vi "R(T) T(t) SETP(t) with ramp332 DC ramp current(File overwrite Fixed)_1.vi"(0 "I":dbl=1e-06 min=1e-09 max=1.0 step=1e-06 format="%.4e", 1 "Ti":dbl min=0.0 max=400.0 format="%.3f", 2 "Tf":dbl=4.0 min=0.0 max=400.0 format="%.3f", 3 "Ramp":ext format="%.3f", 4 "Range":dbl=3.0 format="%.2f", 7 "Measurement":bool=TRUE, 8 "Auto\nTemp?":bool=TRUE) -> ()   [LabVIEW 2012]
panel:
  out "?":cluster{dbl, dbl}[](graph)
  out "?":cluster{"X":dbl, "Y":dbl}[](graph)
  in  "x data precision":i16
  in  "y data precision":i16
  in  "Path":path
  in  "File name":string
  in  "Autorange":bool=TRUE
  in  "Volt Delay":u32=50
  in  "Voltmeter PLC":dbl=1.0 min=0.01 max=60.0 step=0.01 format="%.2f"
  in  "Voltage Compliance":dbl=12.0 min=0.1 max=105.0 step=0.1 format="%.2f"
  in  "minutes to wait before start":u32=5
  out "R/Ohm":dbl=1e-09 min=-1.0 step=1e-09 format="%.3e"
  out "T/K":dbl min=0.0 step=0.01 format="%.3f"
  in  "Delay time":sgl min=0 step=1 format="%.2f"
  # "ON"
  # "OFF"
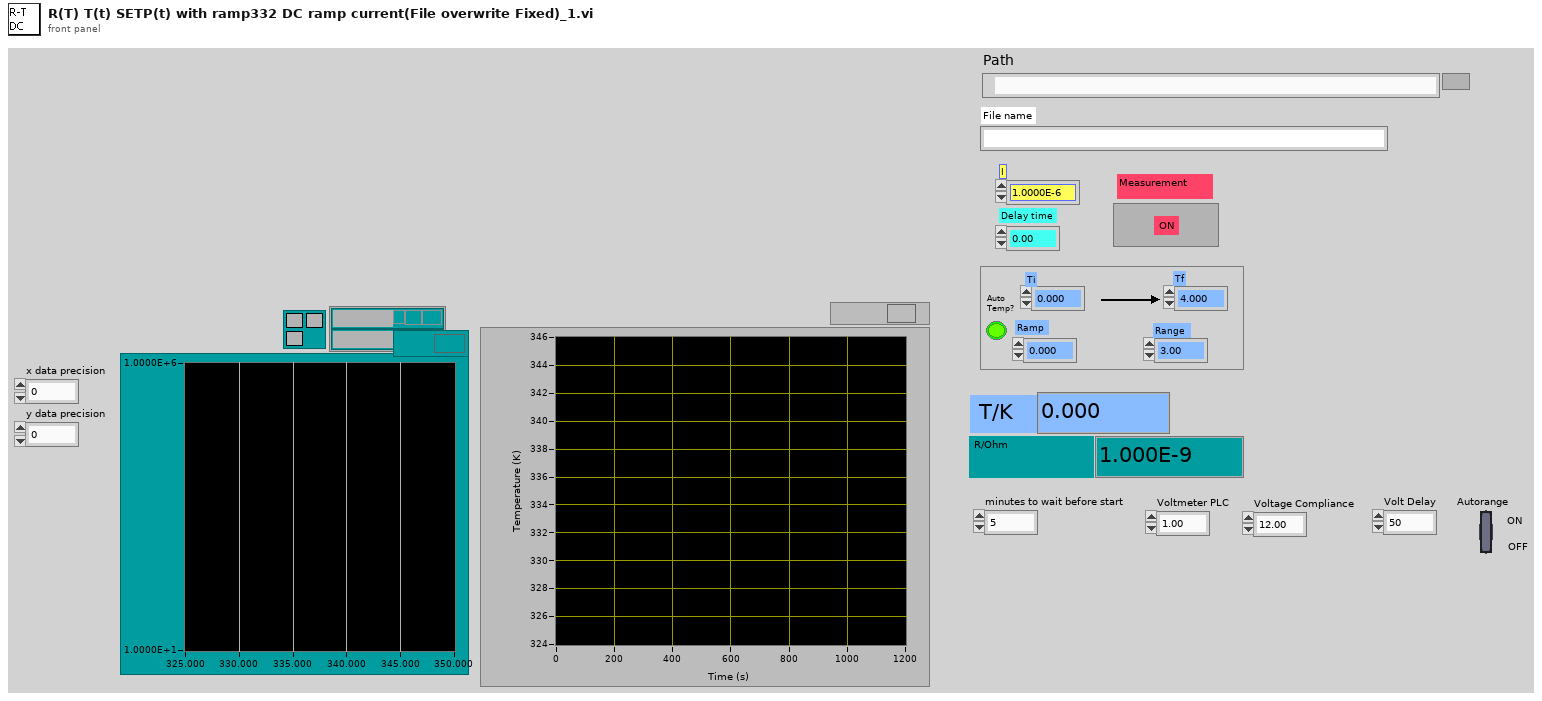
[diagram p1: front panel]
types:
  T1 = enum16{"open", "replace", "create", "open or create", "replace or create", "replace or create with confirmation"}
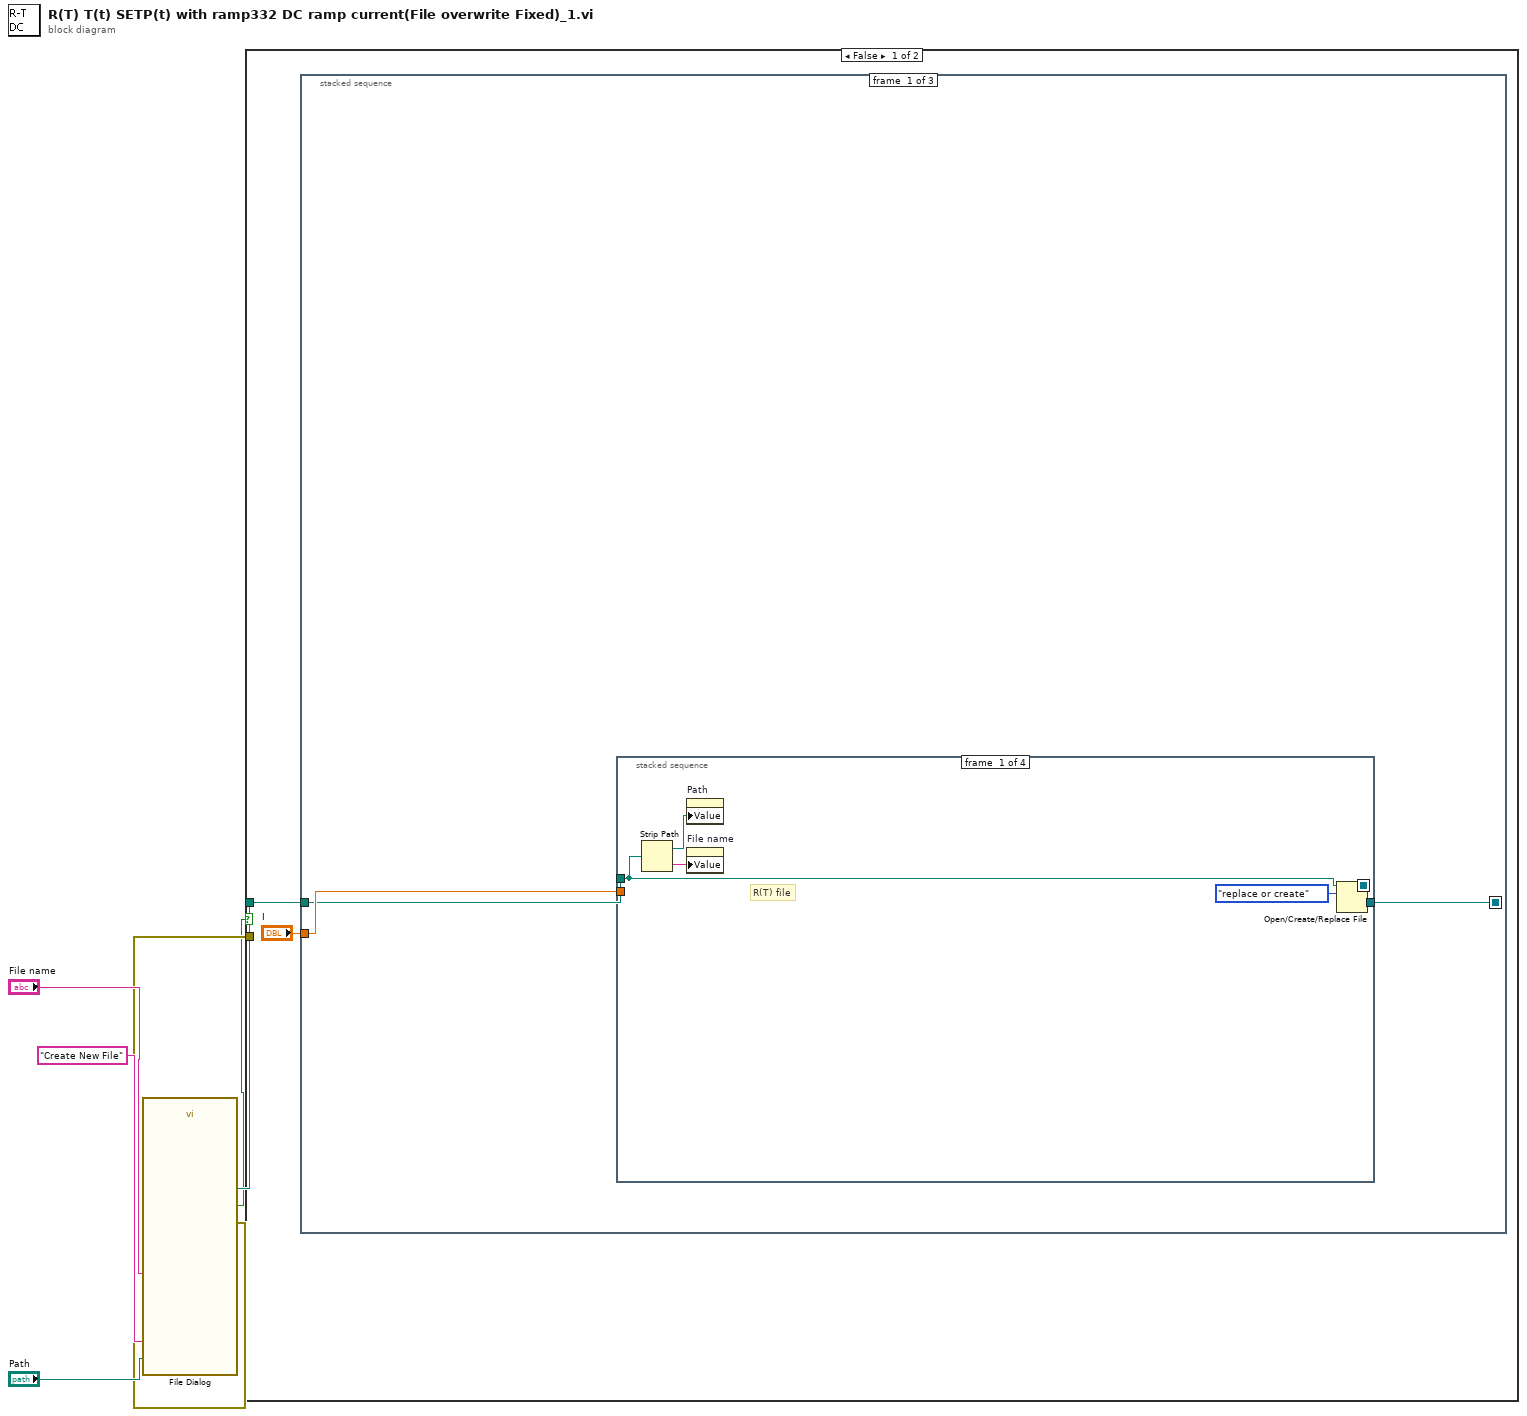
[diagram p0: block diagram]
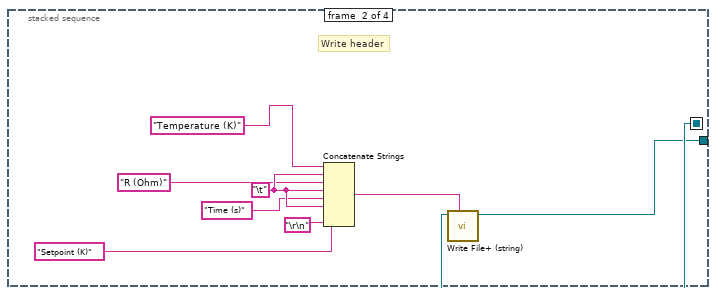
[diagram p2: hidden frame]
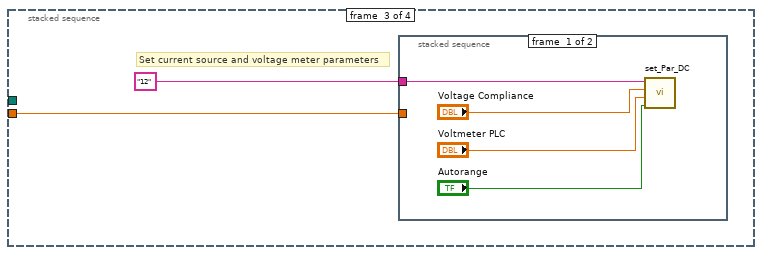
[diagram p3: hidden frame]
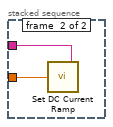
[diagram p4: hidden frame]
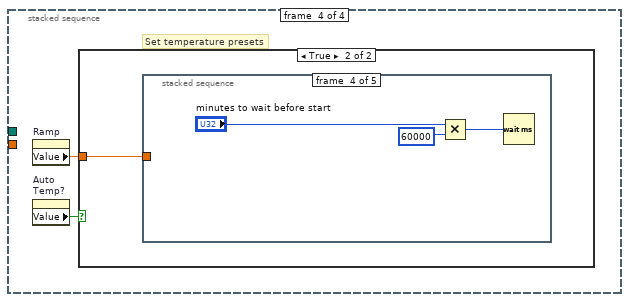
[diagram p5: hidden frame]
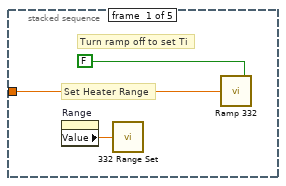
[diagram p7: hidden frame]
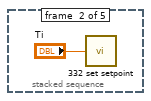
[diagram p8: hidden frame]
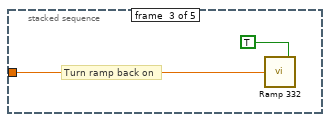
[diagram p9: hidden frame]
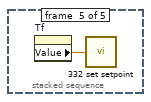
[diagram p10: hidden frame]
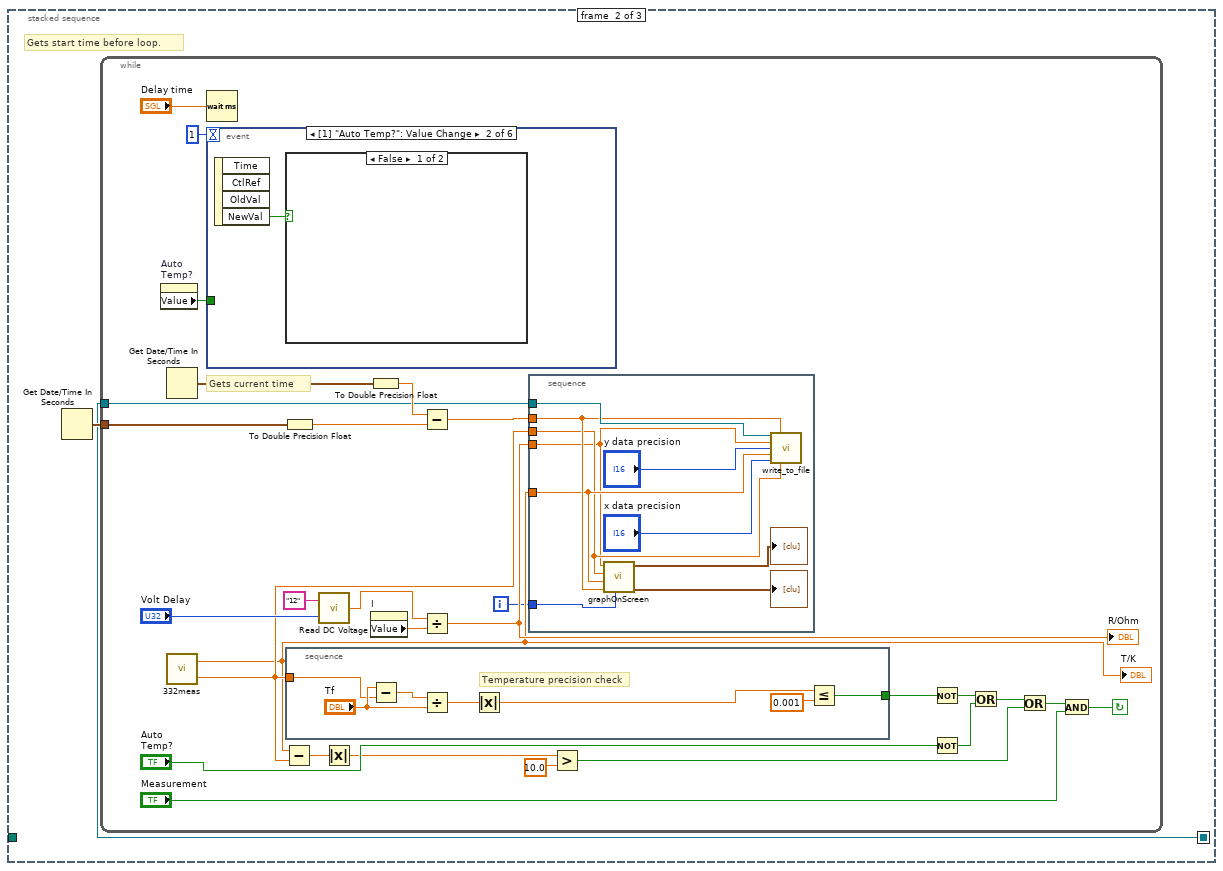
[diagram p11: hidden frame]
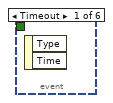
[diagram p12: hidden frame]
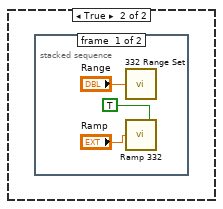
[diagram p13: hidden frame]
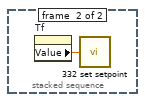
[diagram p14: hidden frame]
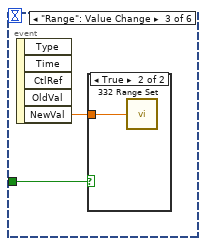
[diagram p15: hidden frame]
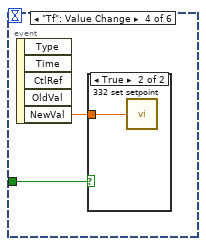
[diagram p17: hidden frame]
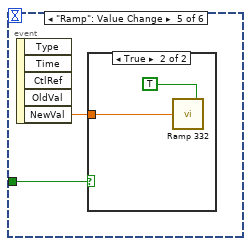
[diagram p19: hidden frame]
diagram:
  n1 = call "File Dialog"("start path"="Path", "prompt"="Create New File", "default name"="File name") -> ("selected path"=w3:path, "cancelled"=w1:bool, "error out"=w2:errorcluster)  [unwired: 9 in, 1 out]
  n2 = case shown="False" w1 {
    tunnel: w3 -> [w8 _]
    tunnel: w2 -> [_ _]
    frame False {
      n3 = stacked-sequence {
        seq-local: [w9 _ _] -> [_ w47 w114]
        tunnel: "I" -> [w11 _ w115]
        tunnel: w8 -> [w10 _ _]
        frame #0 {
          n4 = stacked-sequence {
            seq-local: [w12 _ _ _] -> [_ w22 _ _]
            tunnel: w11 -> [_ _ w26 _]
            tunnel: w10 -> [w13 _ _ _]
            tunnel: [_ w21 _ _] -> w9
            frame #0 {
              # "R(T) file"
              n5 = Strip Path(path=w13) -> (stripped path=w14:path, name=w15:string)
              n6 = property on="Path" class="Path"("Value"=w14) -> ()  [unwired: 2 in, 2 out]
              n7 = property on="File name" class="Str"("Value"=w15) -> ()  [unwired: 2 in, 2 out]
              n8 = Open/Create/Replace File(file path (use dialog)=w13, operation (0:open)=T1."replace or create") -> (refnum out=w12:refnum<file>)  [unwired: 4 in, 2 out]
            }
            frame #1 {
              w24 = "\t"
              # "Write header"
              n9 = Concatenate Strings("Temperature (K)" ("string"), w24, "R (Ohm)" ("string"), w24, "Time (s)" ("string"), w24, "Setpoint (K)" ("string"), "\r\n") -> (w25:string)
              n10 = call <vilib>:"Write File+ (string).vi"("string"=w25, "refnum"=w22) -> ("dup refnum"=w21:refnum<file>)  [unwired: 5 in, 2 out]
            }
            frame #2 {
              # "Set current source and voltage meter parameters"
              n11 = stacked-sequence {
                tunnel: "12" ("Address") -> [w31 w33]
                tunnel: w26 -> [_ w32]
                frame #0 {
                  n12 = call "set_Par_DC.vi"("Autorange"="Autorange", "Voltmeter PLC"="Voltmeter PLC", "Voltage Compliance"="Voltage Compliance", "Address"=w31) -> ()
                }
                frame #1 {
                  n13 = call "Set DC Current Ramp.vi"("Address"=w33, "Current"=w32) -> ()
                }
              }
            }
            frame #3 {
              # "Set temperature presets"
              n14 = property on="Ramp" class="DigNum (strict)"() -> ("Value"=w34:ext)  [unwired: 2 in, 2 out]
              n15 = property on="Auto\nTemp?" class="Bool (strict)"() -> ("Value"=w35:bool)  [unwired: 2 in, 2 out]
              n16 = case shown="True" w35 {
                tunnel: w34 -> [_ w36]
                frame False {
                }
                frame True {
                  n17 = stacked-sequence {
                    tunnel: w36 -> [w38 _ w42 _ _]
                    frame #0 {
                      # "Set Heater Range"
                      # "Turn ramp off to set Ti"
                      n18 = property on="Range" class="DigNum (strict)"() -> ("Value"=w37:dbl)  [unwired: 2 in, 2 out]
                      n19 = call "332 Range Set.vi"("Power Range: 93C\n0=OFF, 1=Low, 2=Med, 3=High"=w37) -> ()
                      n20 = call "Ramp 332.vi"("On"=FALSE, "K/min"=w38) -> ()
                    }
                    frame #1 {
                      n21 = call "332 set setpoint.vi"("Set Temperature SetPoint:332"="Ti") -> ()
                    }
                    frame #2 {
                      # "Turn ramp back on"
                      n22 = call "Ramp 332.vi"("On"=TRUE, "K/min"=w42) -> ()
                    }
                    frame #3 {
                      n23 = Multiply(x="minutes to wait before start", y=u32 60000) -> (x*y=w44:u32)
                      n24 = Wait (ms)(milliseconds to wait=w44) -> ()  [unwired: 1 out]
                    }
                    frame #4 {
                      n25 = property on="Tf" class="DigNum (strict)"() -> ("Value"=w46:dbl)  [unwired: 2 in, 2 out]
                      n26 = call "332 set setpoint.vi"("Set Temperature SetPoint:332"=w46) -> ()
                    }
                  }
                }
              }
            }
          }
        }
        frame #1 {
          # "Gets start time before loop."
          n27 = Get Date/Time In Seconds() -> (seconds since 1Jan1904=w48:timestamp)
          n28 = while {
            tunnel: w48 -> [w61]
            tunnel: w47 -> [w54]
            i -> [w49]
            stop <- w77 continue-if-true
            # "Gets current time"
            n29 = property on="Auto\nTemp?" class="Bool (strict)"() -> ("Value"=w73:bool)  [unwired: 2 in, 2 out]
            n30 = Get Date/Time In Seconds() -> (seconds since 1Jan1904=w63:timestamp)
            n31 = call "332meas.vi"() -> ("332 Temp [K]"=w50:dbl, "332 Temp Setpoint [K]"=w52:dbl)  [unwired: 1 in]
            "T/K" <- w50
            n32 = Wait (ms)(milliseconds to wait="Delay time") -> ()  [unwired: 1 out]
            n33 = event shown="[1] \"Auto Temp?\": Value Change" {
              selector: _ -> [_ _ _ _ _ _]
              dyn-events: _ -> [_ _ _ _ _ _]
              timeout: 1 -> [_ _ _ _ _ _]
              tunnel: w73 -> [_ _ w101 w103 w106 _]
              event Timeout {
                n34 = event-data() -> ()  [unwired: 1 in, 2 out]
              }
              event "Auto\nTemp?": Value Change {
                n35 = event-data() -> ("NewVal"=w95:bool)  [unwired: 1 in, 3 out]
                n36 = case shown="False" w95 {
                  frame False {
                  }
                  frame True {
                    n37 = stacked-sequence {
                      frame #0 {
                        n38 = call "332 Range Set.vi"("Power Range: 93C\n0=OFF, 1=Low, 2=Med, 3=High"="Range") -> ()
                        n39 = call "Ramp 332.vi"("On"=TRUE, "K/min"="Ramp") -> ()
                      }
                      frame #1 {
                        n40 = property on="Tf" class="DigNum (strict)"() -> ("Value"=w99:dbl)  [unwired: 2 in, 2 out]
                        n41 = call "332 set setpoint.vi"("Set Temperature SetPoint:332"=w99) -> ()
                      }
                    }
                  }
                }
              }
              event "Range": Value Change {
                n42 = event-data() -> ("NewVal"=w100:dbl)  [unwired: 1 in, 4 out]
                n43 = case shown="True" w101 {
                  tunnel: w100 -> [_ w102]
                  frame False {
                  }
                  frame True {
                    n44 = call "332 Range Set.vi"("Power Range: 93C\n0=OFF, 1=Low, 2=Med, 3=High"=w102) -> ()
                  }
                }
              }
              event "Tf": Value Change {
                n45 = event-data() -> ("NewVal"=w104:dbl)  [unwired: 1 in, 4 out]
                n46 = case shown="True" w103 {
                  tunnel: w104 -> [_ w105]
                  frame False {
                  }
                  frame True {
                    n47 = call "332 set setpoint.vi"("Set Temperature SetPoint:332"=w105) -> ()
                  }
                }
              }
              event "Ramp": Value Change {
                n48 = event-data() -> ("NewVal"=w107:ext)  [unwired: 1 in, 4 out]
                n49 = case shown="True" w106 {
                  tunnel: w107 -> [_ w108]
                  frame False {
                  }
                  frame True {
                    n50 = call "Ramp 332.vi"("On"=TRUE, "K/min"=w108) -> ()
                  }
                }
              }
              event "I": Value Change {
                n51 = event-data() -> ("NewVal"=w110:dbl)  [unwired: 1 in, 4 out]
                n52 = stacked-sequence {
                  tunnel: w110 -> [_ w112]
                  frame #0 {
                    # "Wait until measurement\nfinished"
                    n53 = Wait (ms)(milliseconds to wait=u32 1000) -> ()  [unwired: 1 out]
                  }
                  frame #1 {
                    n54 = call "Set DC Current.vi"("Address"="24" ("address string"), "Current"=w112) -> ()
                  }
                }
              }
            }
            n55 = Subtract(x=w50, y=w52) -> (x-y=w60:dbl)
            n56 = To Double Precision Float(number=w61) -> (double precision float=w62:dbl)
            n57 = stacked-sequence {
              tunnel: [w89] -> w76
              tunnel: w52 -> [w88]
              frame #0 {
                # "Temperature precision check"
                n58 = Subtract(x="Tf", y=w88) -> (x-y=w92:dbl)
                n59 = Divide(x=w92, y="Tf") -> (x/y=w93:dbl)
                n60 = Absolute Value(x=w93) -> (abs(x)=w91:dbl)
                n61 = Less Or Equal?(x=w91, y=0.001) -> (x <= y?=w89:bool)
              }
            }
            n62 = call "Read DC Voltage.vi"("Volt Delay"="Volt Delay", "Address"="12" ("address string")) -> ("Voltage"=w66:dbl)
            n63 = Absolute Value(x=w60) -> (abs(x)=w56:dbl)
            n64 = To Double Precision Float(number=w63) -> (double precision float=w64:dbl)
            n65 = property on="I" class="DigNum (strict)"() -> ("Value"=w67:dbl)  [unwired: 2 in, 2 out]
            n66 = Subtract(x=w64, y=w62) -> (x-y=w51:dbl)
            n67 = Divide(x=w66, y=w67) -> (x/y=w53:dbl)
            "R/Ohm" <- w53
            n68 = stacked-sequence {
              tunnel: w54 -> [w87]
              tunnel: w53 -> [w78]
              tunnel: w52 -> [w79]
              tunnel: w51 -> [w81]
              tunnel: w50 -> [w80]
              tunnel: w49 -> [w82]
              frame #0 {
                n69 = call "graphOnScreen.vi"("Connect to loop iteration"=w82, "Time"=w81, "332 Temp [K]"=w80, "332 Temp Setpoint [K]"=w79, "R(ohm)"=w78) -> ("T(t)"=→"?":cluster{"X":dbl, "Y":dbl}[], 3:→"?":cluster{dbl, dbl}[])  [unwired: 5 in]
                n70 = call "write_to_file.vi"("refnum"=w87, "Time"=w81, "y data"=w78, "y data precision"="y data precision", "x data"=w80, "x data precision"="x data precision", "Setpoint"=w79) -> ()  [unwired: 8 in, 1 out]
              }
            }
            n71 = Greater?(x=w56, y=10.0) -> (0:w55:bool)
            n72 = Not(x=w76) -> (.not. x?=w74:bool)
            n73 = Not(x="Auto\nTemp?") -> (.not. x?=w69:bool)
            n74 = Or(x=w74, y=w69) -> (x .or. y?=w59:bool)
            n75 = Or(x=w59, y=w55) -> (x .or. y?=w58:bool)
            n76 = And(x=w58, y="Measurement") -> (x .and. y?=w77:bool)
          }
        }
        frame #2 {
          w116 = "12" ("Address")
          n77 = call "Send to Volt Meter.vi"("Address"=w116, "Data"=":trig:sour imm;:init") -> ()
          n78 = stacked-sequence {
            tunnel: w116 -> [w119 w120]
            tunnel: w115 -> [w118 _]
            frame #0 {
              n79 = call "Set DC Current Ramp to Zero.vi"("Address"=w119, "Current"=w118) -> ()
            }
            frame #1 {
              n80 = call "disarm.vi"("address string"=w120) -> ()  [unwired: 1 in, 1 out]
            }
          }
          n81 = Close File(refnum=w114) -> ()  [unwired: 1 in, 2 out]
        }
      }
    }
    frame True {
    }
  }
